vi "Ascii to Hex (1Byte).vi"(2 "Ascii 1":string) -> (0 "Ascii 2":string, 1 "Decimal":u32)   [LabVIEW 2016]
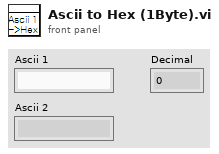
[diagram p1: front panel]
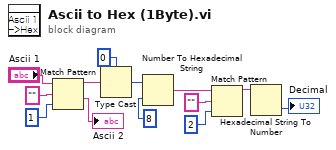
[diagram p0: block diagram]
diagram:
  n1 = Match Pattern(string="Ascii 1", regular expression="" ("정규식"), offset (0)=1 ("길이(나머지)")) -> (before substring=w11:string, after substring=→"Ascii 2":string)  [unwired: 2 out]
  n2 = Type Cast(type=0 ("길이(나머지)"), x=w11) -> (*(type *) &x=w13:i32)
  n3 = Number To Hexadecimal String(1:i16 8 ("폭(-)"), 2:w13) -> (0:w7:string)
  n4 = Match Pattern(string=w7, regular expression="" ("정규식"), offset (0)=2 ("길이(나머지)")) -> (before substring=w2:string)  [unwired: 3 out]
  n5 = Hexadecimal String To Number(string=w2) -> (number=→"Decimal":u32)  [unwired: 2 in, 1 out]
